vi "isWhite.vi"(1 "whiteBOND":dbl) -> (0 "isWhite":bool)   [LabVIEW 2013]
uses:
  <vilib>/NXT/Block Support/NXT_InputPort.ctl
  <vilib>/NXT/Dual Mode Library/Sensors/EV3_Color_Reflect.vi
panel:
  out "Scaled Value":sgl
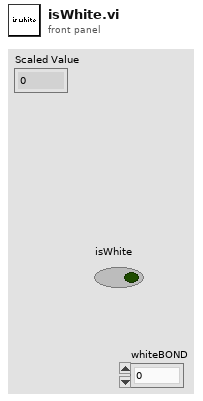
[diagram p1: front panel]
types:
  T1 = typedef "NXT_InputPort.ctl" = u32
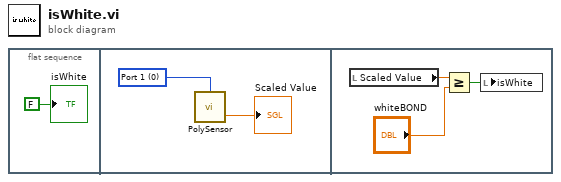
[diagram p0: block diagram]
diagram:
  n1 = flat-sequence {
    frame #0 {
      "isWhite" <- FALSE ("Boolean")
    }
    frame #1 {
      w2 = T1 0 items=["Port 1", "Port 2", "Port 3", "Port 4"] ("Port (Port 1)")
      n2 = call-poly <vilib>:"PolySensor.vi"("Port (Port 1)"=w2) -> ("Scaled Value"=→"Scaled Value":sgl)  [unwired: 2 in, 1 out]
    }
    frame #2 {
      n3 = local read "Scaled Value"() -> (w4:sgl)
      n4 = Greater Or Equal?(x=w4, y="whiteBOND") -> (x >= y?=w5:bool)
      n5 = local write "isWhite"(w5) -> ()
    }
  }
